vi "ProprioceptionThresholding.vi"(1 "Physical Channel(s) 2":tag="Dev1/ao0:3") -> (0 "Prop SR\nThres":dbl)   [LabVIEW 2016]
uses:
  <vilib>/DAQmx/write.llb/DAQmx Write (Analog 1D DBL NChan 1Samp).vi
  <vilib>/DAQmx/create/channels.llb/DAQmx Create Channel (AO-Voltage-Basic).vi
  <vilib>/Utility/inputDevices.llb/keyboardAcquire.vi
  <vilib>/DAQmx/miscellaneous.llb/DAQmx Fill In Error Info.vi
  <vilib>/Utility/inputDevices.llb/closeKeyboard.vi
  <vilib>/Analysis/NI_AALBase.lvlib
panel:
  out "Simulation mode":bool
  in  "Manual Threshold":dbl
  in  "Manually Selected Threshold":bool
  in  "Max Voltage 2":dbl=5.0
  in  "Min Voltage 2":dbl=-5.0
  out "iteration count":i32
  out "Waveform Chart 2":dbl[](graph)
  out "Gauge":dbl(knob) scale=0.0..1.0
  out "Gauge Readings in mV":dbl
  in  "stop 3":bool
  in  "STORE Prop. SR VALUE?":bool
  out "Prop. SR Thresholds":dbl[](array[numeric])
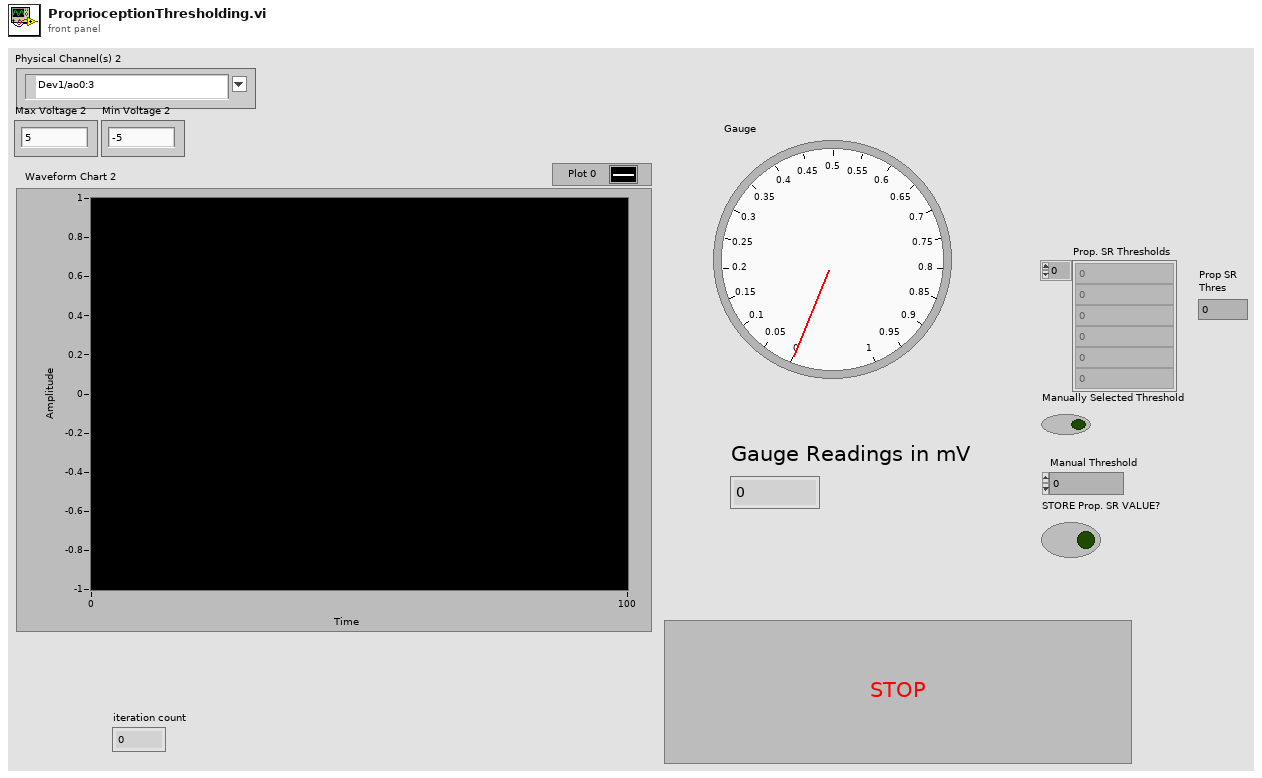
[diagram p1: front panel]
types:
  T1 = enum16{"0", "1", "2", "3", "4", "5", "6", "7", "8", "9", "A", "B", "C", "D", "E", "F", "G", "H", "I", "J", "K", "L", "M", "N", "O", "P", "Q", "R", "S", "T", "U", "V", "W", "X", "Y", "Z", "F1", "F2", "F3", "F4", "F5", "F6", "F7", "F8", "F9", "F10", "F11", "F12", "F13", "F14", "F15", "ADD", "BACK", "BACKSLASH", "CAPITAL", "COMMA", "DECIMAL", "DELETE", "DIVIDE", "DOWN", "END", "EQUALS", "ESCAPE", "GRAVE (`)", "HOME", "INSERT", "LBRACKET", "LCONTROL", "LEFT", "L ALT", "LSHIFT", "LWIN", "MINUS", "MULTIPLY", "NEXT", "NUMLOCK", "NUMPAD_0", "NUMPAD_1", "NUMPAD_2", "NUMPAD_3", "NUMPAD_4", "NUMPAD_5", "NUMPAD_6", "NUMPAD_7", "NUMPAD_8", "NUMPAD_9", "PAUSE", "PERIOD", "PRIOR (PG UP)", "RBRACKET", "RCONTROL", "RETURN", "RIGHT", "R ALT", "RSHIFT", "RWIN", "SCROLL", "SEMICOLON", "SLASH", "SPACE", "SUBTRACT", "TAB", "UP", "ENTER (num pad)", "' (quote)"}[]
  T2 = enum16{"0", "1", "2", "3", "4", "5", "6", "7", "8", "9", "A", "B", "C", "D", "E", "F", "G", "H", "I", "J", "K", "L", "M", "N", "O", "P", "Q", "R", "S", "T", "U", "V", "W", "X", "Y", "Z", "F1", "F2", "F3", "F4", "F5", "F6", "F7", "F8", "F9", "F10", "F11", "F12", "F13", "F14", "F15", "ADD", "BACK", "BACKSLASH", "CAPITAL", "COMMA", "DECIMAL", "DELETE", "DIVIDE", "DOWN", "END", "EQUALS", "ESCAPE", "GRAVE (`)", "HOME", "INSERT", "LBRACKET", "LCONTROL", "LEFT", "L ALT", "LSHIFT", "LWIN", "MINUS", "MULTIPLY", "NEXT", "NUMLOCK", "NUMPAD_0", "NUMPAD_1", "NUMPAD_2", "NUMPAD_3", "NUMPAD_4", "NUMPAD_5", "NUMPAD_6", "NUMPAD_7", "NUMPAD_8", "NUMPAD_9", "PAUSE", "PERIOD", "PRIOR (PG UP)", "RBRACKET", "RCONTROL", "RETURN", "RIGHT", "R ALT", "RSHIFT", "RWIN", "SCROLL", "SEMICOLON", "SLASH", "SPACE", "SUBTRACT", "TAB", "UP", "ENTER (num pad)", "' (quote)"}
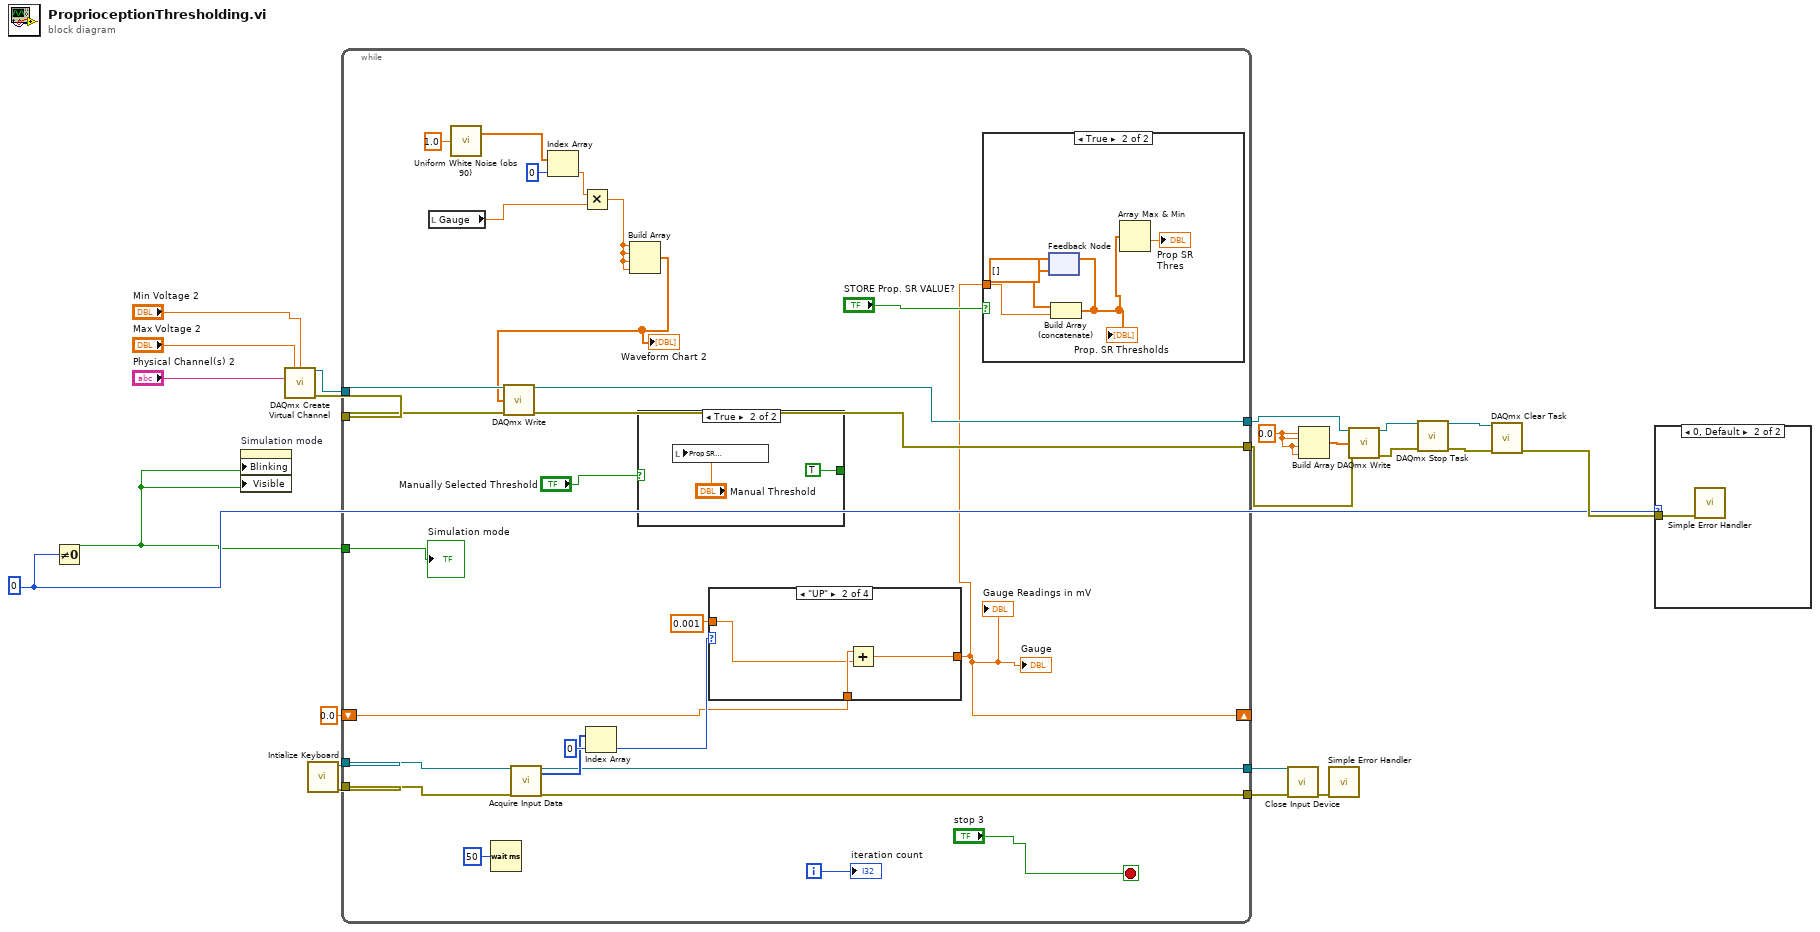
[diagram p0: block diagram]
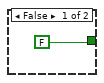
[diagram p3: hidden frame]
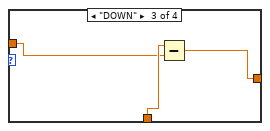
[diagram p6: hidden frame]
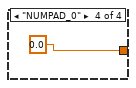
[diagram p7: hidden frame]
diagram:
  w2 = 0
  w3 = 0.0 ("element")
  n1 = Not Equal To 0?(x=w2) -> (x != 0?=w1:bool)
  n2 = property on="Simulation mode" class="Bool (strict)"("Blinking"=w1, "Visible"=w1) -> ()  [unwired: 2 in, 2 out]
  n3 = call-poly <vilib>:"DAQmx Create Virtual Channel.vi"("maximum value"="Max Voltage 2", "minimum value"="Min Voltage 2", "physical channels"="Physical Channel(s) 2") -> ("task out"=w19:refnum<k21>, "error out"=w20:errorcluster)  [unwired: 11 in]
  n4 = call <vilib>:"Intialize Keyboard.vi"() -> ("error out"=w7:errorcluster, "device ID"=w8:refnum<k1>)  [unwired: 10 in]
  n5 = while {
    tunnel: w19 -> [w48]
    tunnel: w20 -> [w47]
    tunnel: [w46] -> w13
    tunnel: [w45] -> w12
    shift-right: [w25] -> _
    shift-left: 0.0 -> [w29]
    tunnel: w8 -> [w37]
    tunnel: w7 -> [w36]
    tunnel: [w33] -> w5
    tunnel: [w32] -> w4
    tunnel: w1 -> [w23]
    i -> [w49]
    stop <- "stop 3" stop-if-true
    n6 = local read "Gauge"() -> (w39:dbl)
    n7 = call <vilib>:"Uniform White Noise (obs 90).vi"("amplitude"=1.0) -> ("uniform white noise"=w42:dbl[])  [unwired: 2 in, 1 out]
    n8 = Wait (ms)(milliseconds to wait=u32 50) -> ()  [unwired: 1 out]
    n9 = call-poly <vilib>:"Acquire Input Data.vi"("device ID"=w37, "error in (no error)"=w36) -> ("device ID"=w33:refnum<k1>, "keys pressed"=w34:T1, "error out"=w32:errorcluster)  [unwired: 15 in]
    n10 = Index Array(array=w42, index=0) -> (element=w40:dbl)
    n11 = Multiply(x=w40, y=w39) -> (x*y=w31:dbl)
    n12 = Index Array(array=w34, index=0) -> (element=w30:T2)
    n13 = Build Array(w31, w31, w31, w31) -> (w38:dbl[])
    "Waveform Chart 2" <- w38
    n14 = call-poly <vilib>:"DAQmx Write.vi"("task/channels in"=w48, "data"=w38, "error in"=w47) -> ("task out"=w46:refnum<k21>, "error out"=w45:errorcluster)  [unwired: 10 in, 1 out]
    n15 = case shown="True" "Manually Selected Threshold" {
      tunnel: [FALSE TRUE] -> _
      frame False {
      }
      frame True {
        n16 = local write "Prop SR\nThres"("Manual Threshold") -> ()
      }
    }
    n17 = case shown="\"UP\"" w30 {
      tunnel: [w58 w61 w64 0.0] -> w25
      tunnel: w29 -> [w58 w60 w63 _]
      tunnel: 0.001 ("step") -> [_ w59 w62 _]
      frame Default {
      }
      frame "UP" {
        n18 = Add(x=w60, y=w59) -> (x+y=w61:dbl)
      }
      frame "DOWN" {
        n19 = Subtract(x=w63, y=w62) -> (x-y=w64:dbl)
      }
      frame "NUMPAD_0" {
      }
    }
    "Gauge" <- w25
    "Gauge Readings in mV" <- w25
    n20 = case shown="True" "STORE Prop. SR VALUE?" {
      tunnel: w25 -> [_ w56]
      frame False {
      }
      frame True {
        n21 = feedback #1(dbl[] []) -> (w57:dbl[])
        n22 = Build Array (concatenate)(w57, w56) -> (w54:dbl[])
        "Prop. SR Thresholds" <- w54
        n23 = feedback-in #1(w54) -> ()
        n24 = Array Max & Min(array=w54) -> (min value=→"Prop SR\nThres":dbl)  [unwired: 3 out]
      }
    }
    "iteration count" <- w49
    "Simulation mode" <- w23
  }
  n25 = call-poly <vilib>:"Close Input Device.vi"("error in (no error)"=w4, "device ID"=w5) -> ("error out"=w6:errorcluster)  [unwired: 8 in]
  n26 = Build Array(w3, w3, w3, w3) -> (w14:dbl[])
  n27 = call <vilib>:"Simple Error Handler.vi"("error in (no error)"=w6) -> ()  [unwired: 4 in, 5 out]
  n28 = call-poly <vilib>:"DAQmx Write.vi"("task/channels in"=w13, "data"=w14, "error in"=w12) -> ("task out"=w16:refnum<k21>, "error out"=w15:errorcluster)  [unwired: 10 in, 1 out]
  n29 = call <vilib>:"DAQmx Stop Task.vi"("task/channels in"=w16, "error in"=w15) -> ("task out"=w18:refnum<k21>, "error out"=w17:errorcluster)  [unwired: 12 in]
  n30 = call <vilib>:"DAQmx Clear Task.vi"("task in"=w18, "error in"=w17) -> ("error out"=w21:errorcluster)  [unwired: 13 in]
  n31 = case shown="0, Default" w2 {
    tunnel: w21 -> [_ w66]
    frame 1 {
    }
    frame 0, Default {
      n32 = call <vilib>:"Simple Error Handler.vi"("error in (no error)"=w66) -> ()  [unwired: 4 in, 5 out]
    }
  }
